vi "Write Range.vi"(8 "error in (no error)":errorcluster, 10 "Range":dbl, 11 "Multimeter in":refnum<class "Multimeter.lvclass">) -> (0 "error out":errorcluster, 3 "Multimeter out":refnum<class "Multimeter.lvclass">)   [LabVIEW 2019, in "Multimeter.lvlib" / "Multimeter.lvclass"]
uses:
  Library/Multimeter.lvclass
  Library/Multimeter.lvclass/Multimeter.ctl
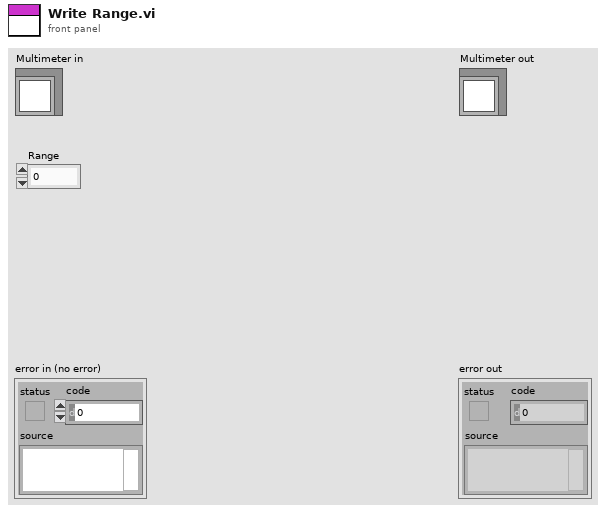
[diagram p1: front panel]
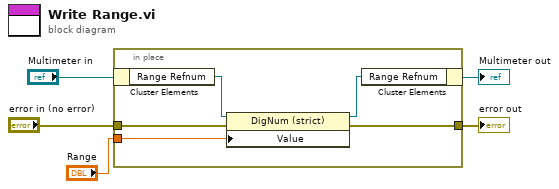
[diagram p0: block diagram]
diagram:
  n1 = in-place {
    in-place-border: [w8] -> w3
    in-place-border: "error in (no error)" -> [w7]
    in-place-border: "Range" -> [w6]
    n2 = in-place-cluster #1("Multimeter in") -> ("Range Refnum"=w10:refnum<vi>)
    n3 = property class="DigNum (strict)"(reference=w10, error in=w7, "Value"=w6) -> (reference out=w9:refnum<vi>, error out=w8:errorcluster)
    n4 = in-place-cluster #1("Range Refnum"=w9) -> (→"Multimeter out":refnum<class "Multimeter.lvclass">)
  }
  "error out" <- w3
